vi "ROI Settings from ini.vi"(7 "Section":string, 8 "error in (no error)":errorcluster, 10 "Operation":T1, 11 "Mask ROI In":T2={"left annulus"={"Center X"=929, "Center Y"=663, "Inner Radius"=200, "Outer Radius"=405, "Start Angle"=90.0, "End Angle"=180.0}, "right annulus"={"Center X"=929, "Center Y"=663, "Inner Radius"=200, "Outer Radius"=405, "Start Angle"=90.0, "End Angle"=180.0}, "Threshold Range"={"Lower value"=106.82432432432432, "Upper value"=255.0}, "[Avg BG]"=[]} {"Threshold Range"."Upper value" min=0.0 max=255.0 scale=0.0..255.0; "Threshold Range"."Lower value" min=0.0 max=255.0 scale=0.0..255.0; "right annulus"."End Angle" format="%.2f"; "right annulus"."Start Angle" format="%.2f"; "right annulus"."Center X" scale=0.0..1024.0; "left annulus"."End Angle" format="%.2f"; "left annulus"."Start Angle" format="%.2f"; "left annulus"."Center X" scale=0.0..1024.0}) -> (0 "error out":errorcluster, 3 "Mask ROI Out":T2={"left annulus"={"Center X"=929, "Center Y"=663, "Inner Radius"=200, "Outer Radius"=405, "Start Angle"=90.0, "End Angle"=180.0}, "right annulus"={"Center X"=929, "Center Y"=663, "Inner Radius"=200, "Outer Radius"=405, "Start Angle"=90.0, "End Angle"=180.0}, "Threshold Range"={"Lower value"=106.82432432432432, "Upper value"=255.0}, "[Avg BG]"=[]} {"Threshold Range"."Upper value" min=0.0 max=255.0 scale=0.0..255.0; "Threshold Range"."Lower value" min=0.0 max=255.0 scale=0.0..255.0; "right annulus"."End Angle" format="%.2f"; "right annulus"."Start Angle" format="%.2f"; "right annulus"."Center X" scale=0.0..1024.0; "left annulus"."End Angle" format="%.2f"; "left annulus"."Start Angle" format="%.2f"; "left annulus"."Center X" scale=0.0..1024.0}, 5 "All Tags Exists?":bool)   [LabVIEW 2013]
doc: "Loads the TCP port being used for listening for incoming connections."
uses:
  Image Processing/Mask ROI Cluster.ctl
  Common/File IO/INI/Read write mode.ctl
  ROI Setting Enum Keys.ctl
  Common/File IO/INI/INI Read write I32.vi
  Common/File IO/INI/INI Read write dbl.vi
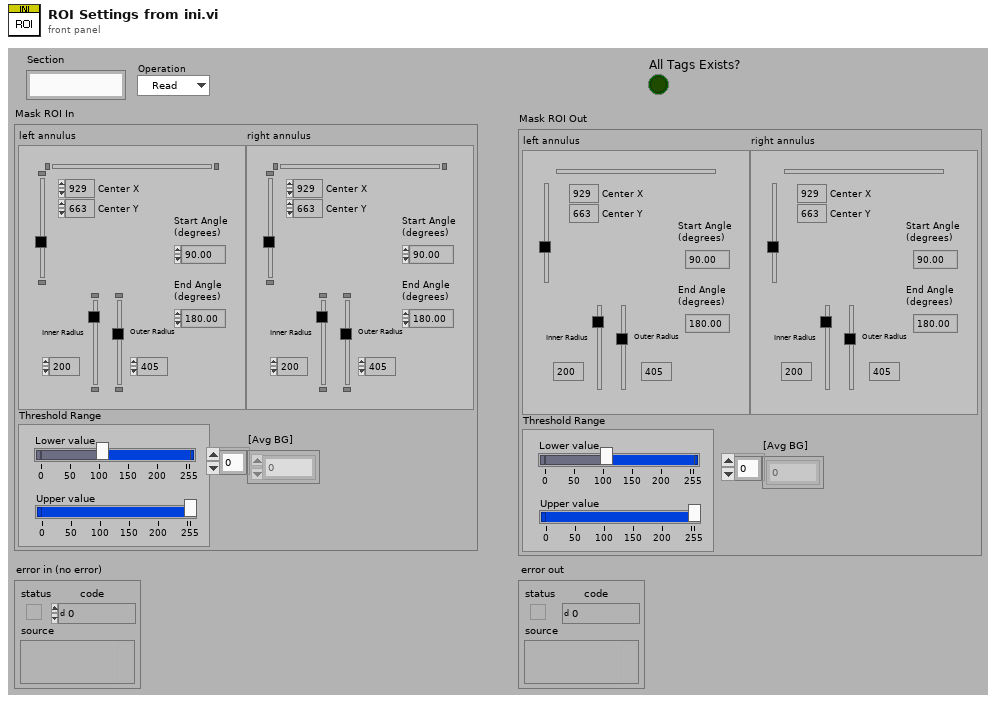
[diagram p1: front panel]
types:
  T1 = typedef "Read write mode.ctl" = enum16{"Read", "Write"}
  T2 = typedef "Mask ROI Cluster.ctl" = cluster{"left annulus":T3, "right annulus":T3, "Threshold Range":cluster{"Lower value":dbl, "Upper value":dbl}, "[Avg BG]":u8[]}
  T3 = typedef "IMAQ Circle" = cluster{"Center X":i32, "Center Y":i32, "Inner Radius":i32, "Outer Radius":i32, "Start Angle":dbl, "End Angle":dbl}
  T4 = typedef "ROI Setting Enum Keys.ctl" = enum16{"Hinge Y", "Hinge X", "Start Angle", "End Angle", "Inner Radius", "Outer Radius", "Lower Threshold", "Sector BG", "Upper Threshold"}
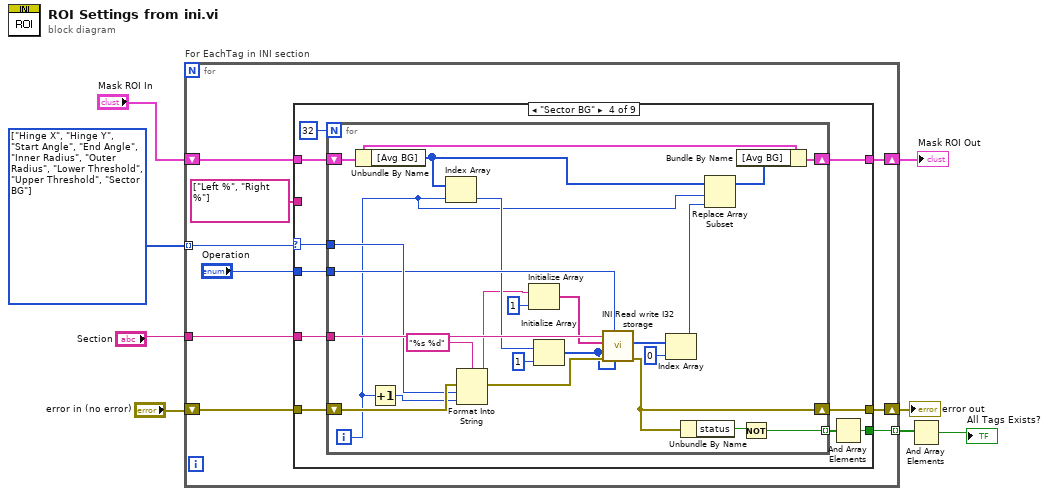
[diagram p0: block diagram]
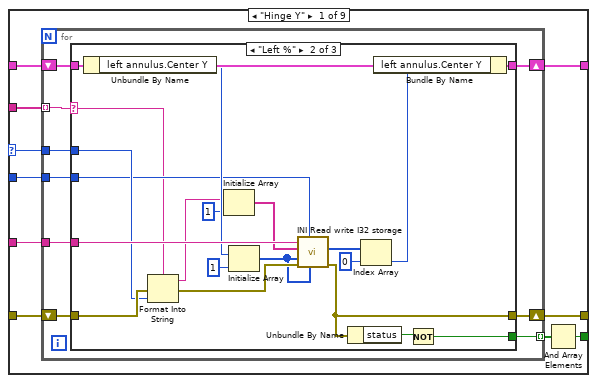
[diagram p2: hidden frame]
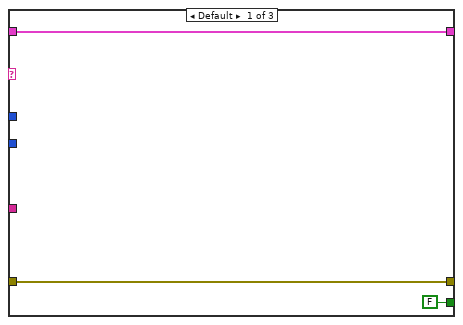
[diagram p3: hidden frame]
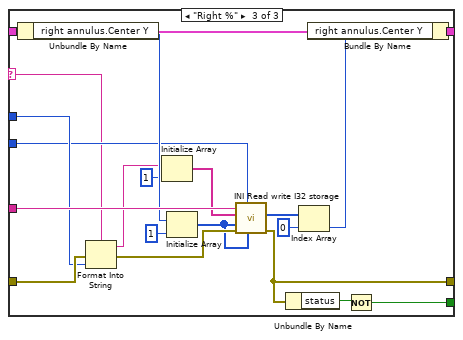
[diagram p4: hidden frame]
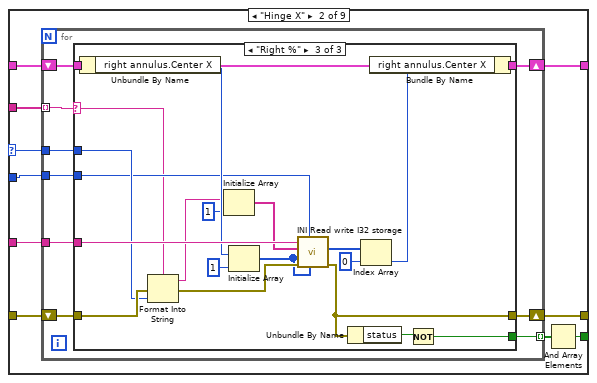
[diagram p5: hidden frame]
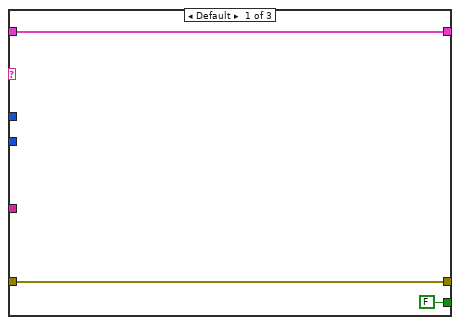
[diagram p6: hidden frame]
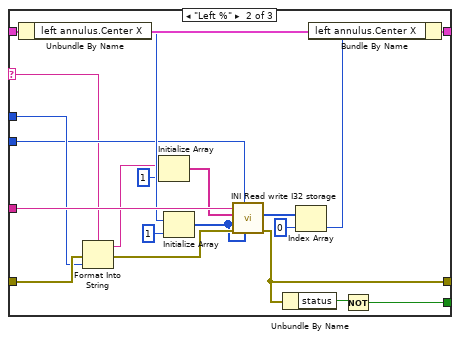
[diagram p7: hidden frame]
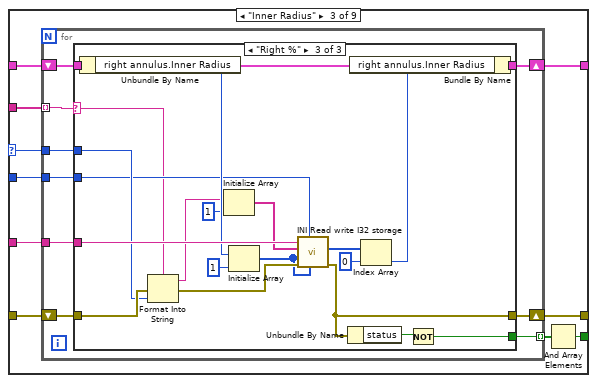
[diagram p8: hidden frame]
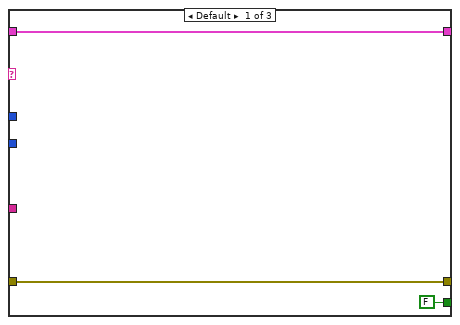
[diagram p9: hidden frame]
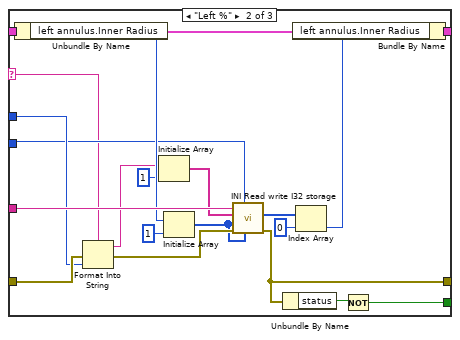
[diagram p10: hidden frame]
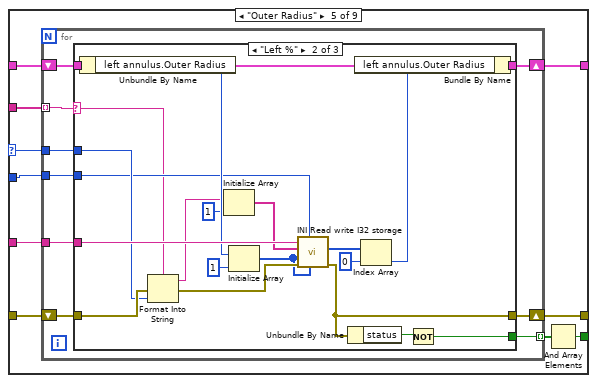
[diagram p11: hidden frame]
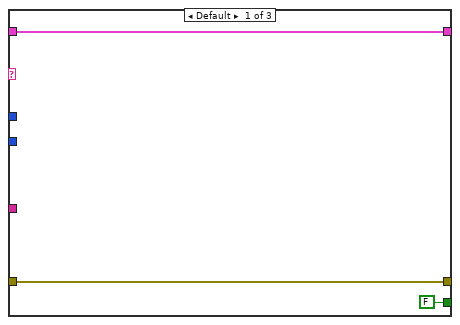
[diagram p12: hidden frame]
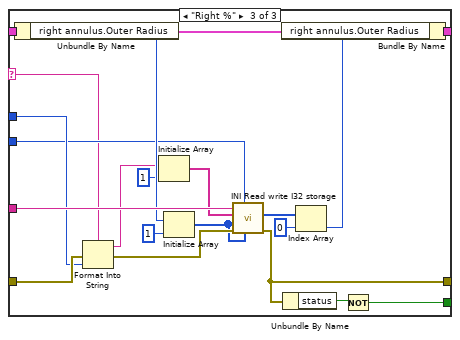
[diagram p13: hidden frame]
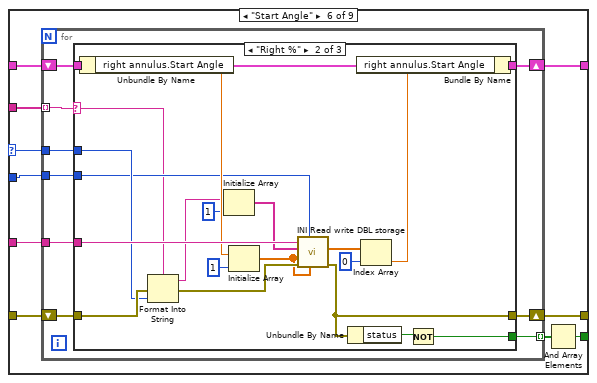
[diagram p14: hidden frame]
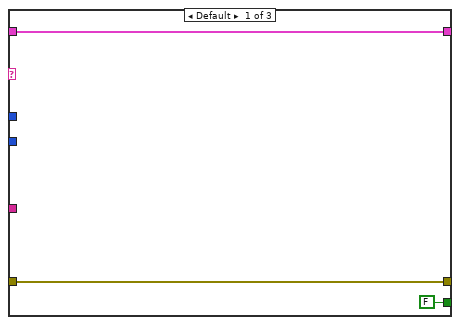
[diagram p15: hidden frame]
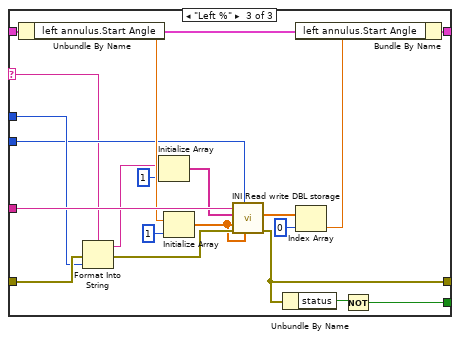
[diagram p16: hidden frame]
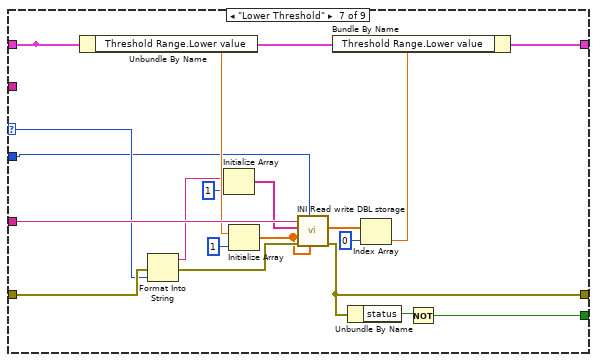
[diagram p17: hidden frame]
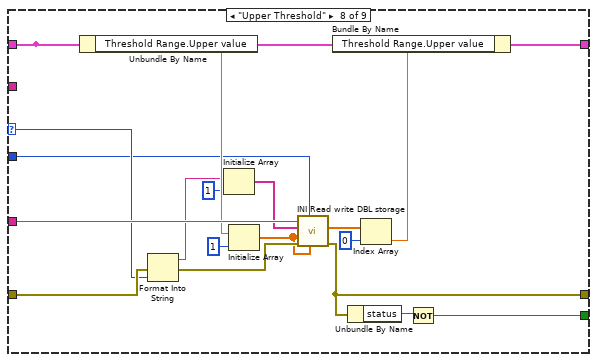
[diagram p18: hidden frame]
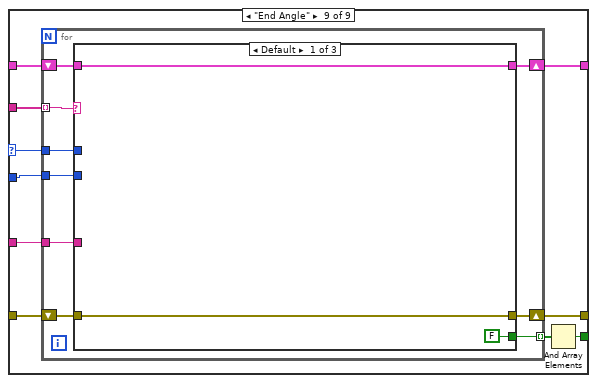
[diagram p19: hidden frame]
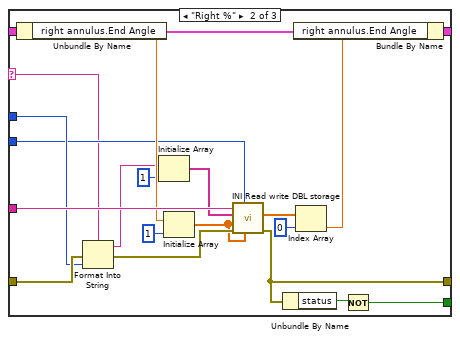
[diagram p20: hidden frame]
diagram:
  w8 = T4[] [enum."Hinge X", enum."Hinge Y", enum."Start Angle", enum."End Angle", enum."Inner Radius", enum."Outer Radius", enum."Lower Threshold", enum."Upper Threshold", enum."Sector BG"] items=["Hinge Y", "Hinge X", "Start Angle", "End Angle", "Inner Radius", "Outer Radius", "Lower Threshold", "Sector BG", "Upper Threshold"]
  n1 = for "For EachTag in INI section" {
    tunnel: "Section" -> [w17]
    tunnel: w8 -> [w11] mode=indexing
    shift-right: [w13] -> w6
    shift-left: "error in (no error)" -> [w15]
    shift-right: [w12] -> w1
    shift-left: "Mask ROI In" -> [w16]
    tunnel: [w14] -> w4 mode=indexing
    n2 = case shown="\"Sector BG\"" w11 {
      selector: w11 -> [w22 w84 w146 w208 w242 w304 w375 w394 w404]
      tunnel: w17 -> [w26 w88 w150 w212 w246 w308 w379 w398 w408]
      tunnel: w16 -> [w24 w86 w148 w210 w244 w306 w377 w396 w406]
      tunnel: w15 -> [w23 w85 w147 w209 w243 w305 w376 w395 w405]
      tunnel: [w27 w89 w151 w213 w247 w309 w380 w399 w409] -> w13
      tunnel: [w19 w81 w143 w206 w239 w301 w364 w383 w401] -> w14
      tunnel: [w25 w87 w149 w211 w245 w307 w378 w397 w407] -> w12
      tunnel: string[] ["Left %", "Right %"] -> [w21 w83 w145 _ w241 w303 _ _ w403]
      tunnel: "Operation" -> [w18 w80 w142 w205 w238 w300 w362 w381 w400]
      frame "Hinge Y" {
        n3 = for {
          tunnel: w26 -> [w35]
          tunnel: w22 -> [w31]
          tunnel: [w30] -> w20 mode=indexing
          shift-right: [w34] -> w25
          shift-left: w24 -> [w33]
          tunnel: w21 -> [w29] mode=indexing
          shift-right: [w36] -> w27
          shift-left: w23 -> [w32]
          tunnel: w18 -> [w28]
          n4 = case shown="\"Left %\"" w29 {
            selector: w29 -> [_ w40 w60]
            tunnel: [w37 w59 w79] -> w36
            tunnel: w35 -> [_ w58 w78]
            tunnel: [w39 w57 w77] -> w34
            tunnel: w33 -> [w39 w56 w76]
            tunnel: w32 -> [w37 w55 w75]
            tunnel: w31 -> [_ w54 w74]
            tunnel: [FALSE w43 w63] -> w30
            tunnel: w28 -> [_ w41 w61]
            frame Default {
            }
            frame "Left %" {
              n5 = Unbundle By Name(w56) -> ("left annulus.Center Y"=w53:i32)
              n6 = Format Into String(format string=w40, error in=w55, w54) -> (resulting string=w51:string, error out=w44:errorcluster)  [unwired: 1 in]
              n7 = Initialize Array(w51, 1 ("dimension size")) -> (w49:string[])
              n8 = Initialize Array(w53, 1 ("dimension size")) -> (w42:i32[])
              n9 = call "INI Read write I32 storage.vi"("Values to write"=w42, "Read/Write mode"=w41, "error in"=w44, "Defaults"=w42, "keys"=w49, "section"=w58) -> ("error out"=w59:errorcluster, "Values"=w48:i32[])  [unwired: 4 in]
              n10 = Unbundle By Name(w59) -> ("status"=w45:bool)
              n11 = Index Array(array=w48, index=0) -> (element=w46:i32)
              n12 = Bundle By Name(cluster=w56, "left annulus.Center Y"=w46) -> (w57:T2)
              n13 = Not(x=w45) -> (.not. x?=w43:bool)
            }
            frame "Right %" {
              n14 = Unbundle By Name(w76) -> ("right annulus.Center Y"=w73:i32)
              n15 = Format Into String(format string=w60, error in=w75, w74) -> (resulting string=w71:string, error out=w64:errorcluster)  [unwired: 1 in]
              n16 = Initialize Array(w71, 1 ("dimension size")) -> (w69:string[])
              n17 = Initialize Array(w73, 1 ("dimension size")) -> (w62:i32[])
              n18 = call "INI Read write I32 storage.vi"("Values to write"=w62, "Read/Write mode"=w61, "error in"=w64, "Defaults"=w62, "keys"=w69, "section"=w78) -> ("error out"=w79:errorcluster, "Values"=w68:i32[])  [unwired: 4 in]
              n19 = Unbundle By Name(w79) -> ("status"=w65:bool)
              n20 = Index Array(array=w68, index=0) -> (element=w66:i32)
              n21 = Bundle By Name(cluster=w76, "right annulus.Center Y"=w66) -> (w77:T2)
              n22 = Not(x=w65) -> (.not. x?=w63:bool)
            }
          }
        }
        n23 = And Array Elements(Boolean array=w20) -> (logical AND=w19:bool)
      }
      frame "Hinge X" {
        n24 = for {
          tunnel: w88 -> [w97]
          tunnel: w84 -> [w93]
          tunnel: [w92] -> w82 mode=indexing
          shift-right: [w96] -> w87
          shift-left: w86 -> [w95]
          tunnel: w83 -> [w91] mode=indexing
          shift-right: [w98] -> w89
          shift-left: w85 -> [w94]
          tunnel: w80 -> [w90]
          n25 = case shown="\"Right %\"" w91 {
            selector: w91 -> [_ w102 w122]
            tunnel: [w99 w121 w141] -> w98
            tunnel: w97 -> [_ w120 w140]
            tunnel: [w101 w119 w139] -> w96
            tunnel: w95 -> [w101 w118 w138]
            tunnel: w94 -> [w99 w117 w137]
            tunnel: w93 -> [_ w116 w136]
            tunnel: [FALSE w105 w125] -> w92
            tunnel: w90 -> [_ w103 w123]
            frame Default {
            }
            frame "Left %" {
              n26 = Unbundle By Name(w118) -> ("left annulus.Center X"=w115:i32)
              n27 = Format Into String(format string=w102, error in=w117, w116) -> (resulting string=w113:string, error out=w106:errorcluster)  [unwired: 1 in]
              n28 = Initialize Array(w113, 1 ("dimension size")) -> (w111:string[])
              n29 = Initialize Array(w115, 1 ("dimension size")) -> (w104:i32[])
              n30 = call "INI Read write I32 storage.vi"("Values to write"=w104, "Read/Write mode"=w103, "error in"=w106, "Defaults"=w104, "keys"=w111, "section"=w120) -> ("error out"=w121:errorcluster, "Values"=w110:i32[])  [unwired: 4 in]
              n31 = Unbundle By Name(w121) -> ("status"=w107:bool)
              n32 = Index Array(array=w110, index=0) -> (element=w108:i32)
              n33 = Bundle By Name(cluster=w118, "left annulus.Center X"=w108) -> (w119:T2)
              n34 = Not(x=w107) -> (.not. x?=w105:bool)
            }
            frame "Right %" {
              n35 = Unbundle By Name(w138) -> ("right annulus.Center X"=w135:i32)
              n36 = Format Into String(format string=w122, error in=w137, w136) -> (resulting string=w133:string, error out=w126:errorcluster)  [unwired: 1 in]
              n37 = Initialize Array(w133, 1 ("dimension size")) -> (w131:string[])
              n38 = Initialize Array(w135, 1 ("dimension size")) -> (w124:i32[])
              n39 = call "INI Read write I32 storage.vi"("Values to write"=w124, "Read/Write mode"=w123, "error in"=w126, "Defaults"=w124, "keys"=w131, "section"=w140) -> ("error out"=w141:errorcluster, "Values"=w130:i32[])  [unwired: 4 in]
              n40 = Unbundle By Name(w141) -> ("status"=w127:bool)
              n41 = Index Array(array=w130, index=0) -> (element=w128:i32)
              n42 = Bundle By Name(cluster=w138, "right annulus.Center X"=w128) -> (w139:T2)
              n43 = Not(x=w127) -> (.not. x?=w125:bool)
            }
          }
        }
        n44 = And Array Elements(Boolean array=w82) -> (logical AND=w81:bool)
      }
      frame "Inner Radius" {
        n45 = for {
          tunnel: w150 -> [w159]
          tunnel: w146 -> [w155]
          tunnel: [w154] -> w144 mode=indexing
          shift-right: [w158] -> w149
          shift-left: w148 -> [w157]
          tunnel: w145 -> [w153] mode=indexing
          shift-right: [w160] -> w151
          shift-left: w147 -> [w156]
          tunnel: w142 -> [w152]
          n46 = case shown="\"Right %\"" w153 {
            selector: w153 -> [_ w164 w184]
            tunnel: [w161 w183 w203] -> w160
            tunnel: w159 -> [_ w182 w202]
            tunnel: [w163 w181 w201] -> w158
            tunnel: w157 -> [w163 w180 w200]
            tunnel: w156 -> [w161 w179 w199]
            tunnel: w155 -> [_ w178 w198]
            tunnel: [FALSE w167 w187] -> w154
            tunnel: w152 -> [_ w165 w185]
            frame Default {
            }
            frame "Left %" {
              n47 = Unbundle By Name(w180) -> ("left annulus.Inner Radius"=w177:i32)
              n48 = Format Into String(format string=w164, error in=w179, w178) -> (resulting string=w175:string, error out=w168:errorcluster)  [unwired: 1 in]
              n49 = Initialize Array(w175, 1 ("dimension size")) -> (w173:string[])
              n50 = Initialize Array(w177, 1 ("dimension size")) -> (w166:i32[])
              n51 = call "INI Read write I32 storage.vi"("Values to write"=w166, "Read/Write mode"=w165, "error in"=w168, "Defaults"=w166, "keys"=w173, "section"=w182) -> ("error out"=w183:errorcluster, "Values"=w172:i32[])  [unwired: 4 in]
              n52 = Unbundle By Name(w183) -> ("status"=w169:bool)
              n53 = Index Array(array=w172, index=0) -> (element=w170:i32)
              n54 = Bundle By Name(cluster=w180, "left annulus.Inner Radius"=w170) -> (w181:T2)
              n55 = Not(x=w169) -> (.not. x?=w167:bool)
            }
            frame "Right %" {
              n56 = Unbundle By Name(w200) -> ("right annulus.Inner Radius"=w197:i32)
              n57 = Format Into String(format string=w184, error in=w199, w198) -> (resulting string=w195:string, error out=w188:errorcluster)  [unwired: 1 in]
              n58 = Initialize Array(w195, 1 ("dimension size")) -> (w193:string[])
              n59 = Initialize Array(w197, 1 ("dimension size")) -> (w186:i32[])
              n60 = call "INI Read write I32 storage.vi"("Values to write"=w186, "Read/Write mode"=w185, "error in"=w188, "Defaults"=w186, "keys"=w193, "section"=w202) -> ("error out"=w203:errorcluster, "Values"=w192:i32[])  [unwired: 4 in]
              n61 = Unbundle By Name(w203) -> ("status"=w189:bool)
              n62 = Index Array(array=w192, index=0) -> (element=w190:i32)
              n63 = Bundle By Name(cluster=w200, "right annulus.Inner Radius"=w190) -> (w201:T2)
              n64 = Not(x=w189) -> (.not. x?=w187:bool)
            }
          }
        }
        n65 = And Array Elements(Boolean array=w144) -> (logical AND=w143:bool)
      }
      frame "Sector BG" {
        n66 = for {
          N: 32 -> [_]
          tunnel: w212 -> [w236]
          tunnel: w208 -> [w232]
          tunnel: [w231] -> w207 mode=indexing
          shift-right: [w235] -> w211
          shift-left: w210 -> [w234]
          shift-right: [w237] -> w213
          shift-left: w209 -> [w233]
          tunnel: w205 -> [w230]
          i -> [w216]
          n67 = Unbundle By Name(w234) -> ("[Avg BG]"=w217:u8[])
          n68 = Increment(x=w216) -> (x+1=w219:i32)
          n69 = Index Array(array=w217, index=w216) -> (element=w221:u8)
          n70 = Format Into String(format string="%s %d", error in=w233, w232, w219) -> (resulting string=w218:string, error out=w223:errorcluster)  [unwired: 1 in]
          n71 = Initialize Array(w218, 1 ("dimension size")) -> (w227:string[])
          n72 = Initialize Array(w221, 1 ("dimension size")) -> (w222:u8[])
          n73 = call "INI Read write I32 storage.vi"("Values to write"=w222, "Read/Write mode"=w230, "error in"=w223, "Defaults"=w222, "keys"=w227, "section"=w236) -> ("error out"=w237:errorcluster, "Values"=w226:i32[])  [unwired: 4 in]
          n74 = Index Array(array=w226, index=0) -> (element=w215:i32)
          n75 = Unbundle By Name(w237) -> ("status"=w224:bool)
          n76 = Replace Array Subset(array=w217, new element=w215, index=w216) -> (w214:u8[])
          n77 = Bundle By Name(cluster=w234, "[Avg BG]"=w214) -> (w235:T2)
          n78 = Not(x=w224) -> (.not. x?=w231:bool)
        }
        n79 = And Array Elements(Boolean array=w207) -> (logical AND=w206:bool)
      }
      frame "Outer Radius" {
        n80 = for {
          tunnel: w246 -> [w255]
          tunnel: w242 -> [w251]
          tunnel: [w250] -> w240 mode=indexing
          shift-right: [w254] -> w245
          shift-left: w244 -> [w253]
          tunnel: w241 -> [w249] mode=indexing
          shift-right: [w256] -> w247
          shift-left: w243 -> [w252]
          tunnel: w238 -> [w248]
          n81 = case shown="\"Left %\"" w249 {
            selector: w249 -> [_ w260 w280]
            tunnel: [w257 w279 w299] -> w256
            tunnel: w255 -> [_ w278 w298]
            tunnel: [w259 w277 w297] -> w254
            tunnel: w253 -> [w259 w276 w296]
            tunnel: w252 -> [w257 w275 w295]
            tunnel: w251 -> [_ w274 w294]
            tunnel: [FALSE w263 w283] -> w250
            tunnel: w248 -> [_ w261 w281]
            frame Default {
            }
            frame "Left %" {
              n82 = Unbundle By Name(w276) -> ("left annulus.Outer Radius"=w273:i32)
              n83 = Format Into String(format string=w260, error in=w275, w274) -> (resulting string=w271:string, error out=w264:errorcluster)  [unwired: 1 in]
              n84 = Initialize Array(w271, 1 ("dimension size")) -> (w269:string[])
              n85 = Initialize Array(w273, 1 ("dimension size")) -> (w262:i32[])
              n86 = call "INI Read write I32 storage.vi"("Values to write"=w262, "Read/Write mode"=w261, "error in"=w264, "Defaults"=w262, "keys"=w269, "section"=w278) -> ("error out"=w279:errorcluster, "Values"=w268:i32[])  [unwired: 4 in]
              n87 = Unbundle By Name(w279) -> ("status"=w265:bool)
              n88 = Index Array(array=w268, index=0) -> (element=w266:i32)
              n89 = Bundle By Name(cluster=w276, "left annulus.Outer Radius"=w266) -> (w277:T2)
              n90 = Not(x=w265) -> (.not. x?=w263:bool)
            }
            frame "Right %" {
              n91 = Unbundle By Name(w296) -> ("right annulus.Outer Radius"=w293:i32)
              n92 = Format Into String(format string=w280, error in=w295, w294) -> (resulting string=w291:string, error out=w284:errorcluster)  [unwired: 1 in]
              n93 = Initialize Array(w291, 1 ("dimension size")) -> (w289:string[])
              n94 = Initialize Array(w293, 1 ("dimension size")) -> (w282:i32[])
              n95 = call "INI Read write I32 storage.vi"("Values to write"=w282, "Read/Write mode"=w281, "error in"=w284, "Defaults"=w282, "keys"=w289, "section"=w298) -> ("error out"=w299:errorcluster, "Values"=w288:i32[])  [unwired: 4 in]
              n96 = Unbundle By Name(w299) -> ("status"=w285:bool)
              n97 = Index Array(array=w288, index=0) -> (element=w286:i32)
              n98 = Bundle By Name(cluster=w296, "right annulus.Outer Radius"=w286) -> (w297:T2)
              n99 = Not(x=w285) -> (.not. x?=w283:bool)
            }
          }
        }
        n100 = And Array Elements(Boolean array=w240) -> (logical AND=w239:bool)
      }
      frame "Start Angle" {
        n101 = for {
          tunnel: w308 -> [w317]
          tunnel: w304 -> [w313]
          tunnel: [w312] -> w302 mode=indexing
          shift-right: [w316] -> w307
          shift-left: w306 -> [w315]
          tunnel: w303 -> [w311] mode=indexing
          shift-right: [w318] -> w309
          shift-left: w305 -> [w314]
          tunnel: w300 -> [w310]
          n102 = case shown="\"Right %\"" w311 {
            selector: w311 -> [_ w322 w342]
            tunnel: [w319 w341 w361] -> w318
            tunnel: w317 -> [_ w340 w360]
            tunnel: [w321 w339 w359] -> w316
            tunnel: w315 -> [w321 w338 w358]
            tunnel: w314 -> [w319 w337 w357]
            tunnel: w313 -> [_ w336 w356]
            tunnel: [FALSE w325 w345] -> w312
            tunnel: w310 -> [_ w323 w343]
            frame Default {
            }
            frame "Right %" {
              n103 = Unbundle By Name(w338) -> ("right annulus.Start Angle"=w335:dbl)
              n104 = Format Into String(format string=w322, error in=w337, w336) -> (resulting string=w333:string, error out=w326:errorcluster)  [unwired: 1 in]
              n105 = Initialize Array(w333, 1 ("dimension size")) -> (w331:string[])
              n106 = Initialize Array(w335, 1 ("dimension size")) -> (w324:dbl[])
              n107 = call "INI Read write DBL storage.vi"("Values to write"=w324, "Read/Write mode"=w323, "error in"=w326, "Default"=w324, "keys"=w331, "section"=w340) -> ("error out"=w341:errorcluster, "Values"=w330:dbl[])  [unwired: 4 in]
              n108 = Unbundle By Name(w341) -> ("status"=w327:bool)
              n109 = Index Array(array=w330, index=0) -> (element=w328:dbl)
              n110 = Bundle By Name(cluster=w338, "right annulus.Start Angle"=w328) -> (w339:T2)
              n111 = Not(x=w327) -> (.not. x?=w325:bool)
            }
            frame "Left %" {
              n112 = Unbundle By Name(w358) -> ("left annulus.Start Angle"=w355:dbl)
              n113 = Format Into String(format string=w342, error in=w357, w356) -> (resulting string=w353:string, error out=w346:errorcluster)  [unwired: 1 in]
              n114 = Initialize Array(w353, 1 ("dimension size")) -> (w351:string[])
              n115 = Initialize Array(w355, 1 ("dimension size")) -> (w344:dbl[])
              n116 = call "INI Read write DBL storage.vi"("Values to write"=w344, "Read/Write mode"=w343, "error in"=w346, "Default"=w344, "keys"=w351, "section"=w360) -> ("error out"=w361:errorcluster, "Values"=w350:dbl[])  [unwired: 4 in]
              n117 = Unbundle By Name(w361) -> ("status"=w347:bool)
              n118 = Index Array(array=w350, index=0) -> (element=w348:dbl)
              n119 = Bundle By Name(cluster=w358, "left annulus.Start Angle"=w348) -> (w359:T2)
              n120 = Not(x=w347) -> (.not. x?=w345:bool)
            }
          }
        }
        n121 = And Array Elements(Boolean array=w302) -> (logical AND=w301:bool)
      }
      frame "Lower Threshold" {
        n122 = Unbundle By Name(w377) -> ("Threshold Range.Lower value"=w374:dbl)
        n123 = Format Into String(error in=w376, w375) -> (resulting string=w372:string, error out=w365:errorcluster)  [unwired: 2 in]
        n124 = Initialize Array(w372, 1 ("dimension size")) -> (w370:string[])
        n125 = Initialize Array(w374, 1 ("dimension size")) -> (w363:dbl[])
        n126 = call "INI Read write DBL storage.vi"("Values to write"=w363, "Read/Write mode"=w362, "error in"=w365, "Default"=w363, "keys"=w370, "section"=w379) -> ("error out"=w380:errorcluster, "Values"=w369:dbl[])  [unwired: 4 in]
        n127 = Unbundle By Name(w380) -> ("status"=w366:bool)
        n128 = Index Array(array=w369, index=0) -> (element=w367:dbl)
        n129 = Bundle By Name(cluster=w377, "Threshold Range.Lower value"=w367) -> (w378:T2)
        n130 = Not(x=w366) -> (.not. x?=w364:bool)
      }
      frame "Upper Threshold" {
        n131 = Unbundle By Name(w396) -> ("Threshold Range.Upper value"=w393:dbl)
        n132 = Format Into String(error in=w395, w394) -> (resulting string=w391:string, error out=w384:errorcluster)  [unwired: 2 in]
        n133 = Initialize Array(w391, 1 ("dimension size")) -> (w389:string[])
        n134 = Initialize Array(w393, 1 ("dimension size")) -> (w382:dbl[])
        n135 = call "INI Read write DBL storage.vi"("Values to write"=w382, "Read/Write mode"=w381, "error in"=w384, "Default"=w382, "keys"=w389, "section"=w398) -> ("error out"=w399:errorcluster, "Values"=w388:dbl[])  [unwired: 4 in]
        n136 = Unbundle By Name(w399) -> ("status"=w385:bool)
        n137 = Index Array(array=w388, index=0) -> (element=w386:dbl)
        n138 = Bundle By Name(cluster=w396, "Threshold Range.Upper value"=w386) -> (w397:T2)
        n139 = Not(x=w385) -> (.not. x?=w383:bool)
      }
      frame "End Angle" {
        n140 = for {
          tunnel: w408 -> [w417]
          tunnel: w404 -> [w413]
          tunnel: [w412] -> w402 mode=indexing
          shift-right: [w416] -> w407
          shift-left: w406 -> [w415]
          tunnel: w403 -> [w411] mode=indexing
          shift-right: [w418] -> w409
          shift-left: w405 -> [w414]
          tunnel: w400 -> [w410]
          n141 = case shown="Default" w411 {
            selector: w411 -> [_ w422 w442]
            tunnel: [w419 w441 w461] -> w418
            tunnel: w417 -> [_ w440 w460]
            tunnel: [w421 w439 w459] -> w416
            tunnel: w415 -> [w421 w438 w458]
            tunnel: w414 -> [w419 w437 w457]
            tunnel: w413 -> [_ w436 w456]
            tunnel: [FALSE w425 w445] -> w412
            tunnel: w410 -> [_ w423 w443]
            frame Default {
            }
            frame "Right %" {
              n142 = Unbundle By Name(w438) -> ("right annulus.End Angle"=w435:dbl)
              n143 = Format Into String(format string=w422, error in=w437, w436) -> (resulting string=w433:string, error out=w426:errorcluster)  [unwired: 1 in]
              n144 = Initialize Array(w433, 1 ("dimension size")) -> (w431:string[])
              n145 = Initialize Array(w435, 1 ("dimension size")) -> (w424:dbl[])
              n146 = call "INI Read write DBL storage.vi"("Values to write"=w424, "Read/Write mode"=w423, "error in"=w426, "Default"=w424, "keys"=w431, "section"=w440) -> ("error out"=w441:errorcluster, "Values"=w430:dbl[])  [unwired: 4 in]
              n147 = Unbundle By Name(w441) -> ("status"=w427:bool)
              n148 = Index Array(array=w430, index=0) -> (element=w428:dbl)
              n149 = Bundle By Name(cluster=w438, "right annulus.End Angle"=w428) -> (w439:T2)
              n150 = Not(x=w427) -> (.not. x?=w425:bool)
            }
            frame "Left %" {
              n151 = Unbundle By Name(w458) -> ("left annulus.End Angle"=w455:dbl)
              n152 = Format Into String(format string=w442, error in=w457, w456) -> (resulting string=w453:string, error out=w446:errorcluster)  [unwired: 1 in]
              n153 = Initialize Array(w453, 1 ("dimension size")) -> (w451:string[])
              n154 = Initialize Array(w455, 1 ("dimension size")) -> (w444:dbl[])
              n155 = call "INI Read write DBL storage.vi"("Values to write"=w444, "Read/Write mode"=w443, "error in"=w446, "Default"=w444, "keys"=w451, "section"=w460) -> ("error out"=w461:errorcluster, "Values"=w450:dbl[])  [unwired: 4 in]
              n156 = Unbundle By Name(w461) -> ("status"=w447:bool)
              n157 = Index Array(array=w450, index=0) -> (element=w448:dbl)
              n158 = Bundle By Name(cluster=w458, "left annulus.End Angle"=w448) -> (w459:T2)
              n159 = Not(x=w447) -> (.not. x?=w445:bool)
            }
          }
        }
        n160 = And Array Elements(Boolean array=w402) -> (logical AND=w401:bool)
      }
    }
  }
  "error out" <- w6
  "Mask ROI Out" <- w1
  n161 = And Array Elements(Boolean array=w4) -> (logical AND=→"All Tags Exists?":bool)
